vi "历史温度曲线.vi"() -> ()   [LabVIEW 2016, in "斯坦道总磷.lvlib"]
uses:
  <vilib>/Utility/miscctls.llb/LVPointTypeDef.ctl
  <vilib>/Utility/miscctls.llb/LVRowAndColumnUnsignedTypeDef.ctl
  <vilib>/Utility/tdmsutil.llb/TDMSFileViewerLocalizedText.vi
panel:
  in  "参数下拉列表":u16(ring) items=["总氮"=2]
  out "名称":string
  in  "选项卡控件":enum32{"趋势图", "测试数据"}(tab)
  out "波形图":waveform(dbl)[](graph)
  out "显示值":string
  in  "多列列表框":i32(listbox)
  in  "列表框":i32(listbox)
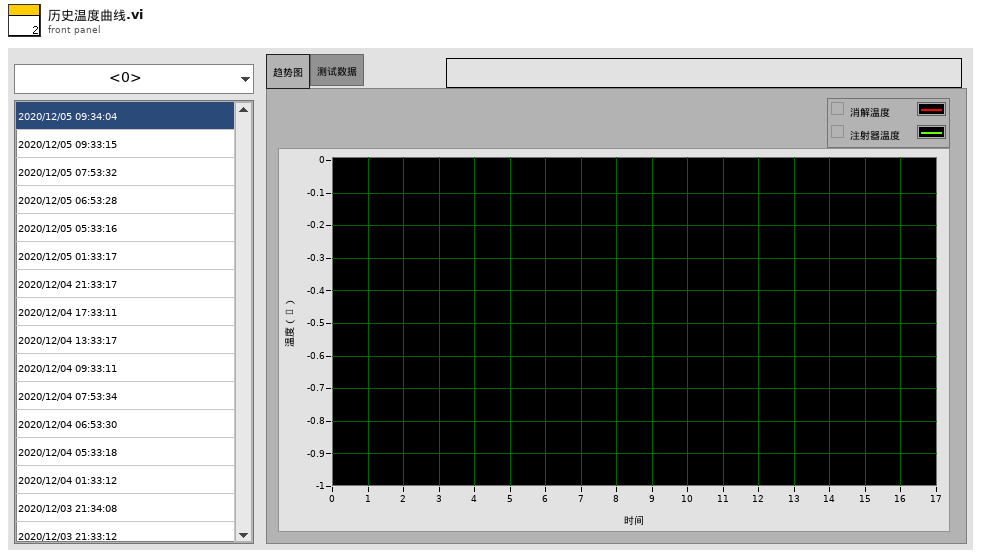
[diagram p1: front panel]
types:
  T1 = typedef "LVRowAndColumnUnsignedTypeDef.ctl" = cluster{"Row":u32, "Column":u32}
  T2 = typedef "LVPointTypeDef.ctl" = cluster{"Horizontal":i16, "Vertical":i16}
  T3 = typedef "LVStringsAndValuesArrayTypeDef_U16.ctl" = cluster{"String":string, "Value":u16}[]
  T4 = typedef "LVPoint32TypeDef.ctl" = cluster{"Horizontal":i32, "Vertical":i32}
  T5 = typedef "Type Enum.ctl" = enum8{"Void", "I8", "I16", "I32", "I64", "U8", "U16", "U32", "U64", "Single Float", "Double Float", "Extended Float", "Single Complex", "Double Complex", "Extended Complex", "Enum I8 NEVER", "Enum I16 NEVER", "Enum I32 NEVER", "Enum I64 NEVER", "Enum U8", "Enum U16", "Enum U32", "Enum U64", "Single Float With Unit", "Double Float With Unit", "Extended Float With Unit", "Single Complex With Unit", "Double Complex With Unit", "Extended Complex With Unit", "boolU16", "Boolean", "String", "Handle", "Path", "Picture", "C String", "Pascal String", "Tag", "SubString", "Array", "SubArray", "Cluster", "Numeric Cluster", "Variant", "LV Variant", "Measure Data (waveform)", "Refnum", "ExtData", "function", "Typedef", "Poly VI", "bad wire", "LabVIEW Class Instance"}
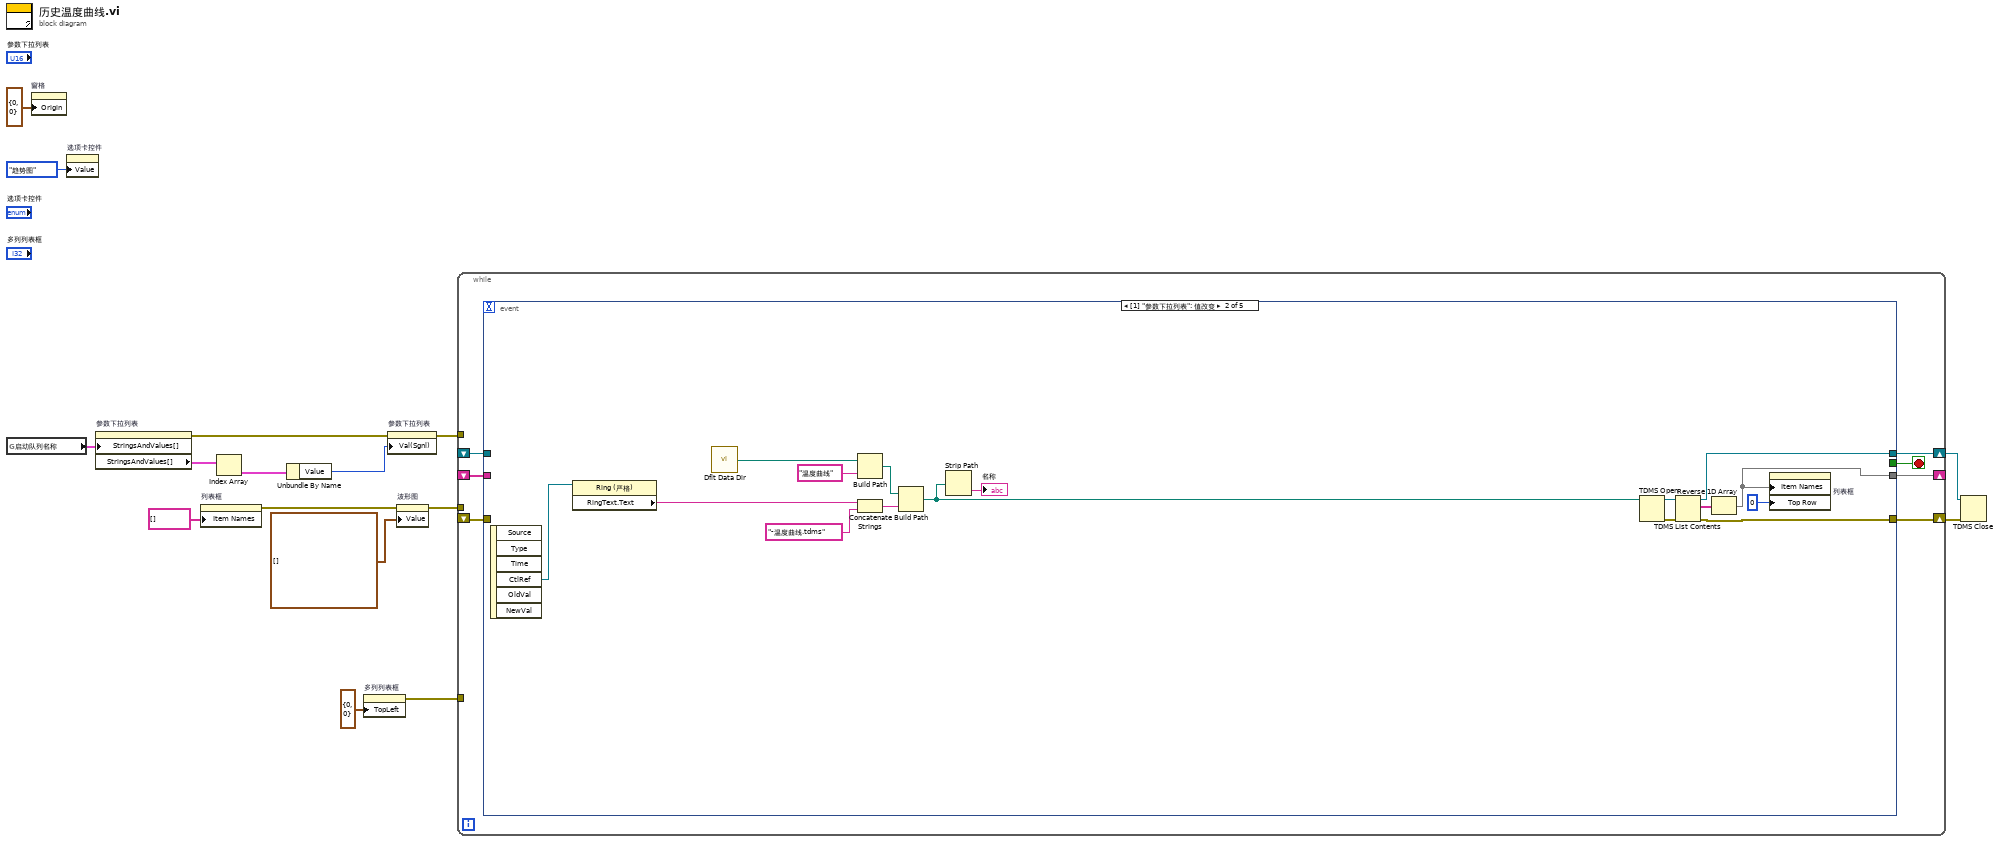
[diagram p0: block diagram]
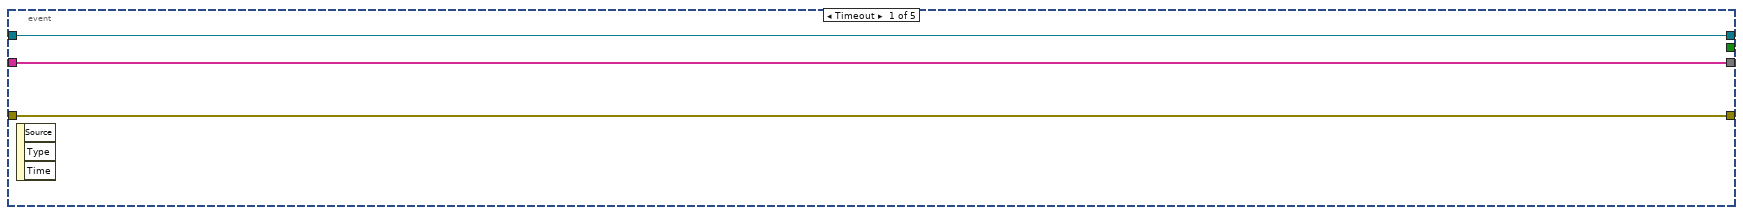
[diagram p2: hidden frame]
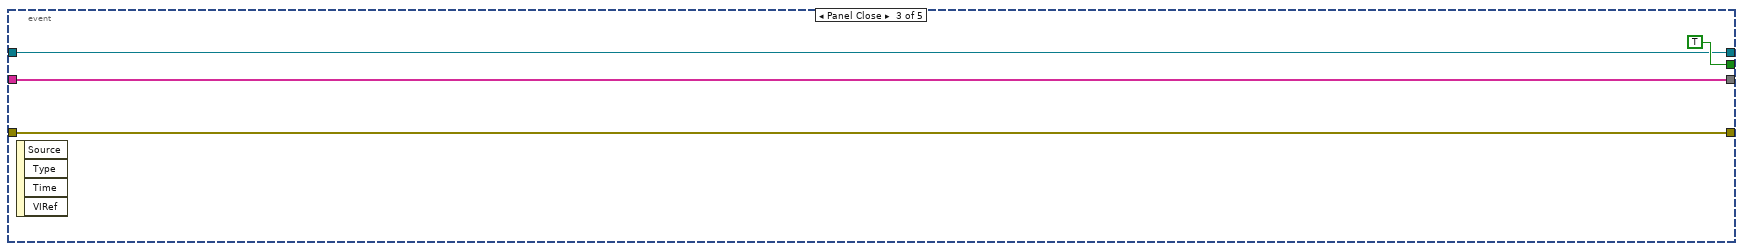
[diagram p3: hidden frame]
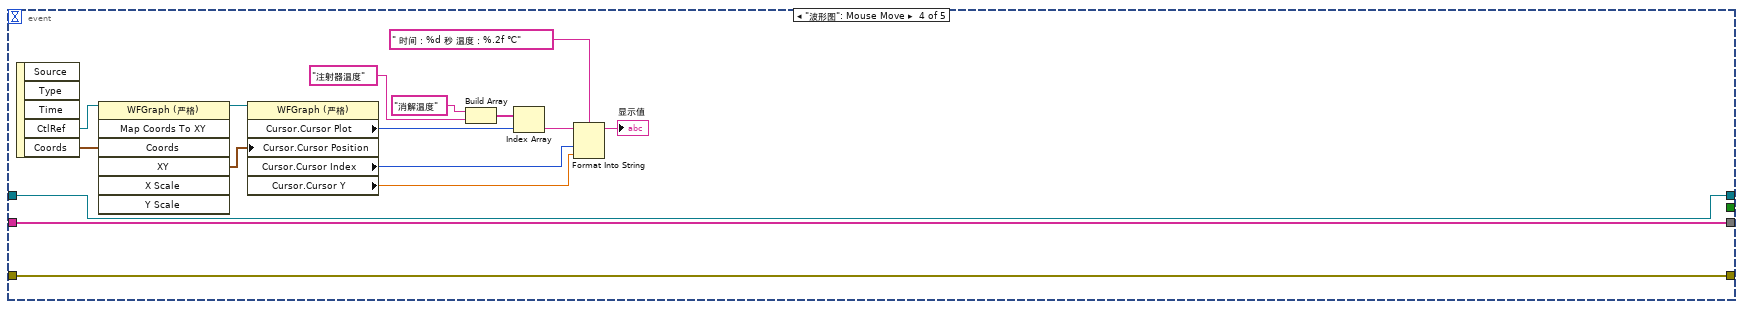
[diagram p4: hidden frame]
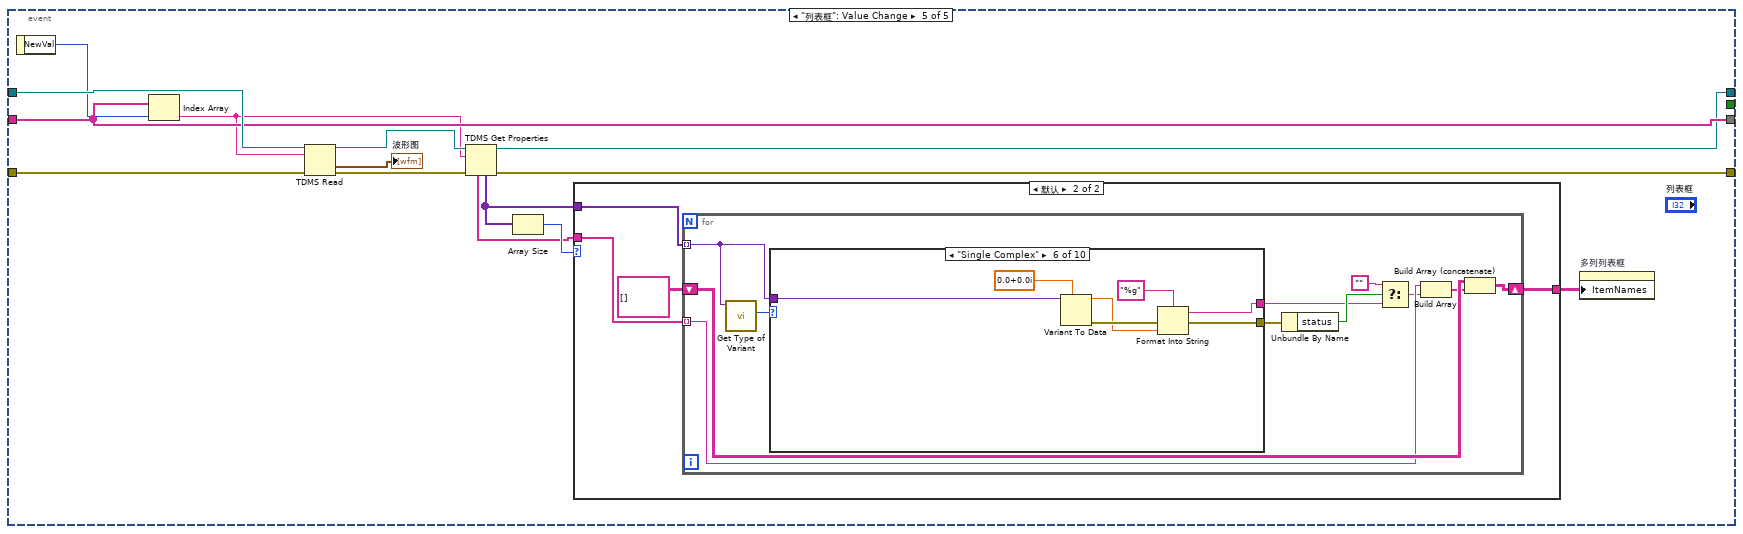
[diagram p5: hidden frame]
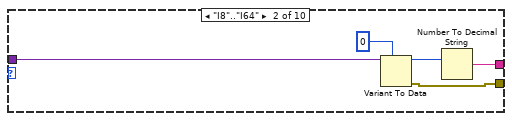
[diagram p8: hidden frame]
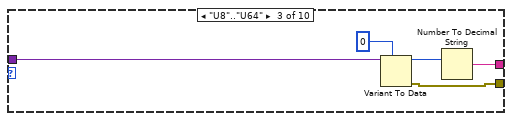
[diagram p9: hidden frame]
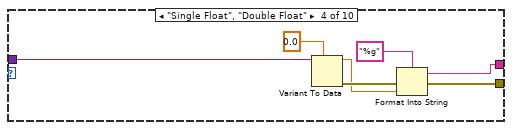
[diagram p10: hidden frame]
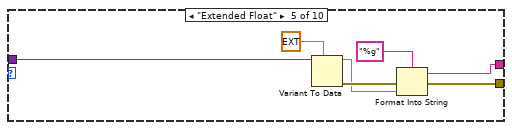
[diagram p11: hidden frame]
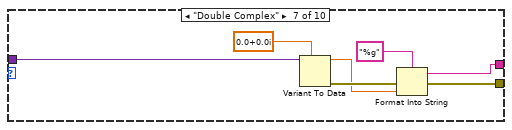
[diagram p12: hidden frame]
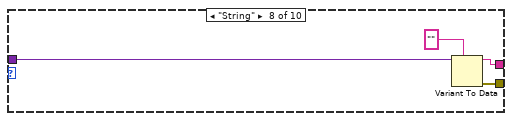
[diagram p13: hidden frame]
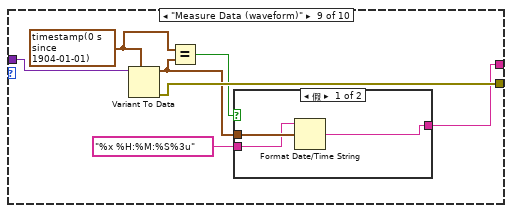
[diagram p14: hidden frame]
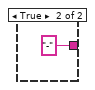
[diagram p15: hidden frame]
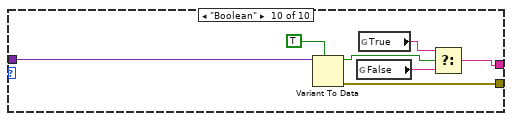
[diagram p16: hidden frame]
diagram:
  n1 = global read "总磷总氮断电保存全局变量.vi" "启动队列名称"() -> (w4:cluster{"String":string, "Value":u16}[])
  n2 = property on="窗格" class="Pane"("Origin"=T2 {"Horizontal"=0, "Vertical"=0} ("原点")) -> ()  [unwired: 2 in, 2 out]
  n3 = property on="选项卡控件" class="TabCtl (严格)"("Value"=enum32{"趋势图", "测试数据"}."趋势图" ("选项卡控件")) -> ()  [unwired: 2 in, 2 out]
  n4 = property on="参数下拉列表" class="Ring (严格)"("StringsAndValues[]"=w4) -> (error out=w7:errorcluster, "StringsAndValues[]"=w5:T3)  [unwired: 2 in, 1 out]
  n5 = property on="列表框" class="LstBox (严格)"("Item Names"=string[] [] ("项名")) -> (error out=w13:errorcluster)  [unwired: 2 in, 1 out]
  n6 = Index Array(array=w5) -> (element=w6:cluster{"String":string, "Value":u16})  [unwired: 1 in]
  n7 = Unbundle By Name(w6) -> ("Value"=w8:u16)
  n8 = property on="多列列表框" class="MCListbox (严格)"("TopLeft"=T1 {"Row"=0, "Column"=0} ("左上可见单元格")) -> (error out=w2:errorcluster)  [unwired: 2 in, 1 out]
  n9 = property on="参数下拉列表" class="Ring (严格)"(error in=w7, "Val(Sgnl)"=w8) -> (error out=w3:errorcluster)  [unwired: 1 in, 1 out]
  n10 = property on="波形图" class="WFGraph (严格)"(error in=w13, "Value"=waveform(dbl)[] [] ("波形图")) -> (error out=w9:errorcluster)  [unwired: 1 in, 1 out]
  n11 = while {
    shift-right: [w21] -> w12
    shift-left: _ -> [w23]
    shift-right: [w20] -> w11
    shift-left: _ -> [w22]
    tunnel: w9 -> [_]
    shift-right: [w17] -> _
    shift-left: _ -> [w19]
    tunnel: w3 -> [_]
    tunnel: w2 -> [_]
    stop <- w18 stop-if-true
    n12 = event shown="[1] \"参数下拉列表\": 值改变" {
      selector: _ -> [_ _ _ _ _]
      dyn-events: _ -> [_ _ _ _ _]
      timeout: _ -> [_ _ _ _ _]
      tunnel: w23 -> [w26 _ w45 w59 w76]
      tunnel: w22 -> [w25 _ w44 w58 w75]
      tunnel: [w26 w34 w45 w59 w65] -> w21
      tunnel: [w25 w33 w44 w58 w64] -> w20
      tunnel: w19 -> [w24 _ w43 w47 w74]
      tunnel: [_ _ TRUE _ _] -> w18
      tunnel: [w24 w27 w43 w47 w74] -> w17
      event Timeout {
        n13 = event-data() -> ()  [unwired: 1 in, 3 out]
      }
      event "参数下拉列表": Value Change {
        n14 = event-data() -> ("CtlRef"=w32:refnum<vi>)  [unwired: 1 in, 5 out]
        n15 = property class="Ring (严格)"(reference=w32) -> ("RingText.Text"=w30:string)  [unwired: 1 in, 2 out]
        n16 = call <vilib>:"Dflt Data Dir.vi"() -> ("App:Default Data Directory"=w35:path)
        n17 = Build Path(base path=w35, name or relative path="温度曲线" ("名称或相对路径")) -> (appended path=w37:path)
        n18 = Concatenate Strings(w30, "-温度曲线.tdms" ("字符串")) -> (w29:string)
        n19 = Build Path(base path=w37, name or relative path=w29) -> (appended path=w38:path)
        n20 = Strip Path(path=w38) -> (name=→"名称":string)  [unwired: 1 out]
        n21 = TDMS Open(11:w38) -> (0:w40:errorcluster, 3:w39:refnum<k34>)  [unwired: 6 in]
        n22 = TDMS List Contents(4:w40, 7:w39) -> (0:w33:errorcluster, 2:w41:string[], 3:w34:refnum<k34>)  [unwired: 1 in, 1 out]
        n23 = Reverse 1D Array(array=w41) -> (reversed array=w27:string[])
        n24 = property on="列表框" class="LstBox (严格)"("Item Names"=w27, "Top Row"=0 ("顶行")) -> ()  [unwired: 2 in, 2 out]
      }
      event Panel Close {
        n25 = event-data() -> ()  [unwired: 1 in, 4 out]
      }
      event "波形图": Mouse Move {
        n26 = event-data() -> ("CtlRef"=w57:refnum<vi>, "Coords"=w56:T4)  [unwired: 1 in, 3 out]
        n27 = invoke on="调用节点" class="WFGraph (严格)" method="Map Coords To XY"(reference=w57, "Coords"=w56) -> (reference out=w54:refnum<vi>, "XY"=w62:cluster{"X":dbl, "Y":dbl})  [unwired: 5 in, 5 out]
        n28 = property on="属性节点" class="WFGraph (严格)"(reference=w54, "Cursor.Cursor Position"=w62) -> ("Cursor.Cursor Plot"=w52:i32, "Cursor.Cursor Index"=w60:i32, "Cursor.Cursor Y"=w53:dbl)  [unwired: 1 in, 2 out]
        n29 = Build Array("消解温度", "注射器温度") -> (w49:string[])
        n30 = Index Array(array=w49, index=w52) -> (element=w48:string)
        n31 = Format Into String(format string=" 时间：%d 秒 温度：%.2f ℃" ("格式字符串"), initial string=w48, w60, w53) -> (resulting string=→"显示值":string)  [unwired: 1 in, 1 out]
      }
      event "列表框": Value Change {
        n32 = event-data() -> ("NewVal"=w73:i32)  [unwired: 1 in]
        n33 = Index Array(array=w74, index=w73) -> (element=w67:string)
        n34 = TDMS Read(0:w76, 5:w67, 11:w75) -> (4:w68:refnum<k34>, 10:→"波形图":waveform(dbl)[], 15:w66:errorcluster)  [unwired: 5 in, 3 out]
        n35 = TDMS Get Properties(8:w66, 10:w67, 11:w68) -> (0:w64:errorcluster, 3:w65:refnum<k34>, 4:w69:variant[], 6:w70:string[])  [unwired: 3 in, 2 out]
        n36 = Array Size(array=w69) -> (size(s)=w71:i32)
        n37 = case shown="默认" w71 {
          tunnel: w70 -> [_ w80]
          tunnel: w69 -> [_ w79]
          tunnel: [_ w77] -> w63
          frame 0 {
          }
          frame Default {
            n38 = for {
              tunnel: w79 -> [w91] mode=indexing
              tunnel: w80 -> [w88] mode=indexing
              shift-right: [w89] -> w77
              shift-left: string[][] [] -> [w90]
              n39 = call <vilib>:"Get Type of Variant.vi"("Data In"=w91) -> ("Type Enum"=w87:T5)  [unwired: 9 in, 1 out]
              n40 = case shown="\"Single Complex\"" w87 {
                tunnel: w91 -> [_ w96 w101 w108 w115 w122 w129 w133 w140 w151]
                tunnel: [_ w93 w98 w105 w111 w118 w126 w131 w139 w150] -> w86
                tunnel: [_ w92 w97 w104 w110 w119 w125 w130 w138 w147] -> w84
                frame "Void", Default {
                }
                frame "I8".."I64" {
                  n41 = Variant To Data(type=i64 0 ("offset (0)"), Variant=w96) -> (data=w94:i64, error out=w93:errorcluster)  [unwired: 1 in]
                  n42 = Number To Decimal String(number=w94) -> (decimal integer string=w92:string)  [unwired: 1 in]
                }
                frame "U8".."U64" {
                  n43 = Variant To Data(type=u64 0 ("offset (0)"), Variant=w101) -> (data=w99:u64, error out=w98:errorcluster)  [unwired: 1 in]
                  n44 = Number To Decimal String(number=w99) -> (decimal integer string=w97:string)  [unwired: 1 in]
                }
                frame "Single Float", "Double Float" {
                  n45 = Variant To Data(type=0.0 ("offset (0)"), Variant=w108) -> (data=w102:dbl, error out=w106:errorcluster)  [unwired: 1 in]
                  n46 = Format Into String(format string="%g", error in=w106, w102) -> (resulting string=w104:string, error out=w105:errorcluster)  [unwired: 1 in]
                }
                frame "Extended Float" {
                  n47 = Variant To Data(type=ext 0.0 ("offset (0)"), Variant=w115) -> (data=w109:ext, error out=w112:errorcluster)  [unwired: 1 in]
                  n48 = Format Into String(format string="%g", error in=w112, w109) -> (resulting string=w110:string, error out=w111:errorcluster)  [unwired: 1 in]
                }
                frame "Single Complex" {
                  n49 = Variant To Data(type=csg 0.0+0.0i, Variant=w122) -> (data=w117:csg, error out=w120:errorcluster)  [unwired: 1 in]
                  n50 = Format Into String(format string="%g", error in=w120, w117) -> (resulting string=w119:string, error out=w118:errorcluster)  [unwired: 1 in]
                }
                frame "Double Complex" {
                  n51 = Variant To Data(type=cdb 0.0+0.0i, Variant=w129) -> (data=w124:cdb, error out=w127:errorcluster)  [unwired: 1 in]
                  n52 = Format Into String(format string="%g", error in=w127, w124) -> (resulting string=w125:string, error out=w126:errorcluster)  [unwired: 1 in]
                }
                frame "String" {
                  n53 = Variant To Data(type="" ("offset (0)"), Variant=w133) -> (data=w130:string, error out=w131:errorcluster)  [unwired: 1 in]
                }
                frame "Measure Data (waveform)" {
                  w137 = timestamp(0 s since 1904-01-01) ("offset (0)")
                  n54 = Variant To Data(type=w137, Variant=w140) -> (data=w136:timestamp, error out=w139:errorcluster)  [unwired: 1 in]
                  n55 = Equal?(x=w137, y=w136) -> (x = y?=w135:bool)
                  n56 = case shown="假" w135 {
                    tunnel: w136 -> [w143 _]
                    tunnel: [w142 "-" ("date/time string")] -> w138
                    tunnel: "%x %H:%M:%S%3u" ("time format string (%c)") -> [w141 _]
                    frame False {
                      n57 = Format Date/Time String(time format string (%c)=w141, seconds (now)=w143) -> (date/time string=w142:string)  [unwired: 1 in]
                    }
                    frame True {
                    }
                  }
                }
                frame "Boolean" {
                  n58 = Variant To Data(type=TRUE, Variant=w151) -> (data=w148:bool, error out=w150:errorcluster)  [unwired: 1 in]
                  n59 = global read "TDMSFileViewerLocalizedText.vi" "False"() -> (w146:string)
                  n60 = global read "TDMSFileViewerLocalizedText.vi" "True"() -> (w145:string)
                  n61 = Select(t=w145, s=w148, f=w146) -> (s? t:f=w147:string)
                }
              }
              n62 = Unbundle By Name(w86) -> ("status"=w85:bool)
              n63 = Select(t="", s=w85, f=w84) -> (s? t:f=w82:string)
              n64 = Build Array(w88, w82) -> (w81:string[])
              n65 = Build Array (concatenate)(w90, w81) -> (w89:string[][])
            }
          }
        }
        n66 = property on="多列列表框" class="MCListbox (严格)"("ItemNames"=w63) -> ()  [unwired: 2 in, 2 out]
      }
    }
  }
  n67 = TDMS Close(8:w11, 11:w12) -> ()  [unwired: 2 out]
